vi "NI AO_test.vi"() -> ()   [LabVIEW 2019]
uses:
  <vilib>/Utility/error.llb/DialogType.ctl
  <vilib>/DAQmx/write.llb/DAQmx Write (Analog 1D Wfm NChan NSamp).vi
  <vilib>/DAQmx/create/channels.llb/DAQmx Create Channel (AO-Voltage-Basic).vi
  <vilib>/DAQmx/configure/timing.llb/DAQmx Timing (Sample Clock).vi
  <vilib>/DAQmx/configure/trigger.llb/DAQmx Start Trigger (Digital Edge).vi
  <vilib>/DAQmx/configure/trigger.llb/DAQmx Start Trigger (Time).vi
  <vilib>/DAQmx/configure/trigger.llb/DAQmx Start Trigger (Analog Edge).vi
  <vilib>/DAQmx/miscellaneous.llb/DAQmx Fill In Error Info.vi
  <resource>/objmgr/daqmx.rc
  <vilib>/measure/NI_MABase.lvlib
panel:
  in  "off time":dbl
  in  "offset":dbl=3.0 format="%#_13g"
  out "x-y":dbl
  in  "stop":bool
  in  "square wave duty cycle (%)":dbl=50.0 format="%0.2f"
  in  "Trigger Type":T1(tab)
  in  "Digital Start Trigger Edge":i32(ring)=10280 caption="Edge" items=["Rising"=10280, "Falling"=10171]
  in  "Digital Start Trigger Source":tag="/Dev1/PFI0" caption="Source"
  in  "Digital Pause Trigger Pause When":i32(ring)=10192 caption="Pause When" items=["High"=10192, "Low"=10214]
  in  "Digital Pause Trigger Source":tag="/Dev1/PFI0" caption="Source"
  in  "Analog Start Trigger Level":dbl caption="Level" format="%0.2f"
  in  "Analog Start Trigger Hysteresis":dbl caption="Hysteresis" format="%.2f"
  in  "Analog Start Trigger Slope":i32(ring)=10280 caption="Slope" items=["Rising"=10280, "Falling"=10171]
  in  "Analog Start Trigger Source":string="APFI0" caption="Source"
  in  "Analog Pause Trigger Source":string="APFI0" caption="Source"
  in  "Analog Pause Trigger Pause When":i32(ring)=10093 caption="Pause When" items=["Above Level"=10093, "Below Level"=10107]
  in  "Analog Pause Trigger Level":dbl caption="Level" format="%.2f"
  in  "When":timestamp
  in  "Select Time\nManually":bool
  out "Waveform Graph":waveform(dbl)[](graph)=[{"t0"=timestamp(0 s since 1904-01-01), "dt"=0.001, "Y"=[]}]
  in  "Output Array":T2(array[cluster])=[{"Waveform Type"=0, "Amplitude"=1.0, "Frequency"=10.0}] {"Frequency" format="%0.2p"; "Amplitude" format="%0.2p"; "Waveform Type" items=["Sine Wave", "Triangle Wave", "Square Wave", "Sawtooth Wave"]}
  in  "Number of Samples":i32=1000
  in  "Sample Rate":dbl=1000.0
  in  "Sample Clock Source":tag="OnboardClock"
  in  "Max Voltage":dbl=5.0
  in  "Min Voltage":dbl=-5.0
  in  "Physical Channel(s)":tag="Dev1/ao0"
  out "Actual Sample Rate":dbl=1000.0 format="%0.2f"
  # "To enable triggers, select a tab above, and configure the settings.\n\nNot all hardware supports all trigger types. Refer to your device documentation for more information."
  # "This trigger type is not supported in output tasks. \n\nRefer to your device documentation for more information on which triggers are supported."
  # "This trigger type is not supported in output tasks. \n\nRefer to your device documentation for more information on which triggers are supported."
  # "If time is not manually set, task will begin after 10 seconds"
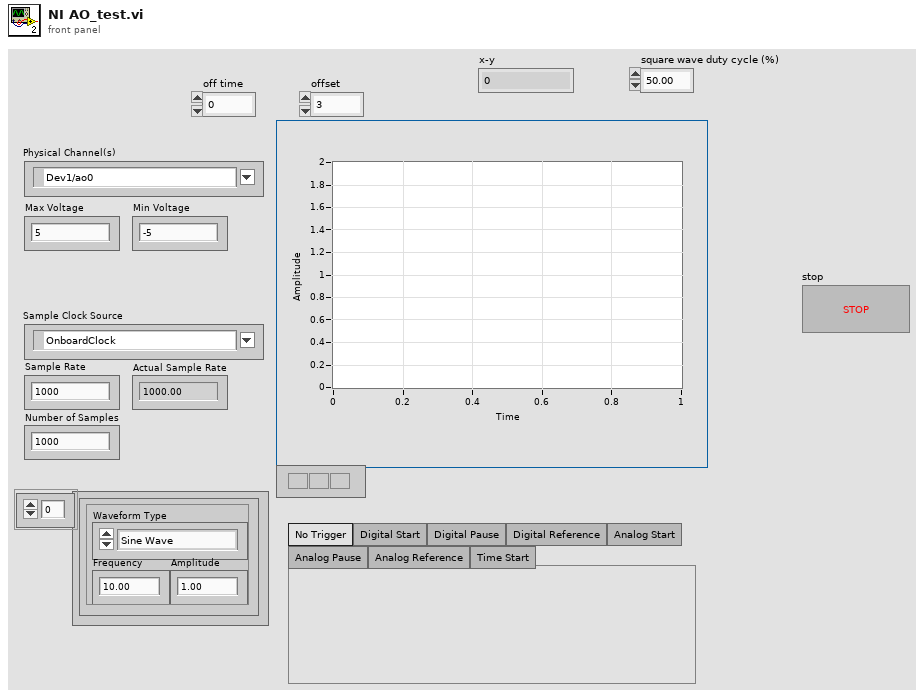
[diagram p1: front panel]
types:
  T1 = enum32{"No Trigger", "Digital Start", "Digital Pause", "Digital Reference", "Analog Start", "Analog Pause", "Analog Reference", "Time Start"}
  T2 = cluster{"Waveform Type":u16, "Amplitude":dbl, "Frequency":dbl}[]
  T3 = typedef "DialogType.ctl" = u16
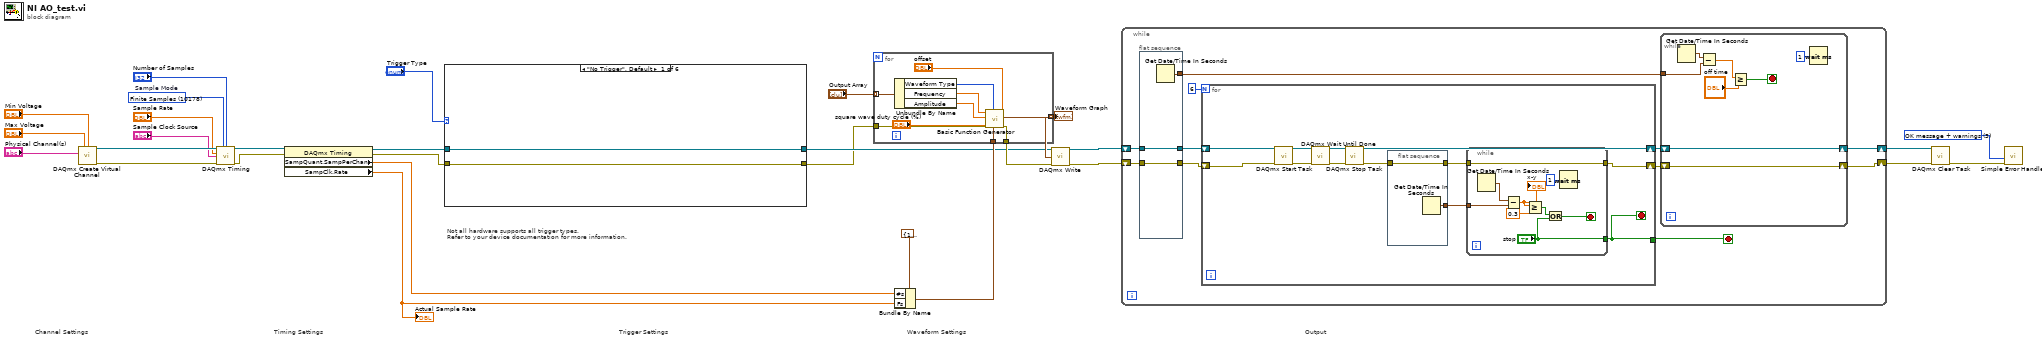
[diagram p0: block diagram]
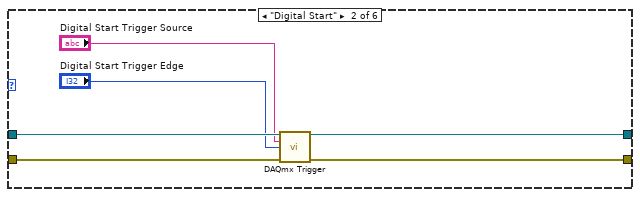
[diagram p2: hidden frame]
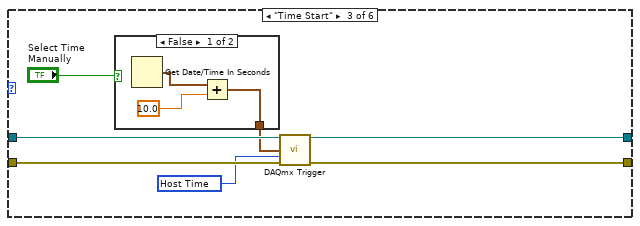
[diagram p3: hidden frame]
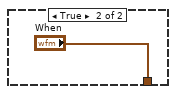
[diagram p4: hidden frame]
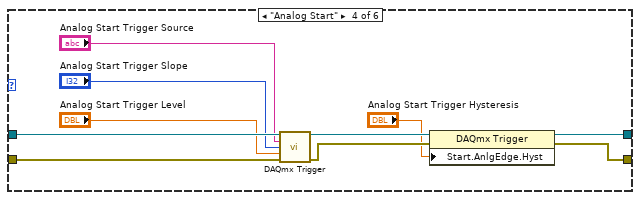
[diagram p5: hidden frame]
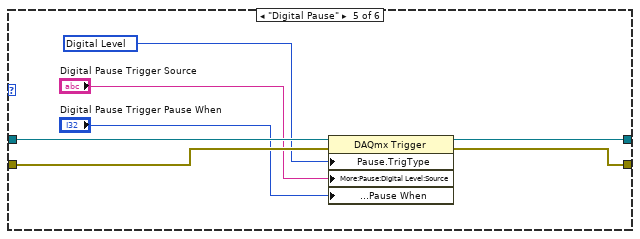
[diagram p6: hidden frame]
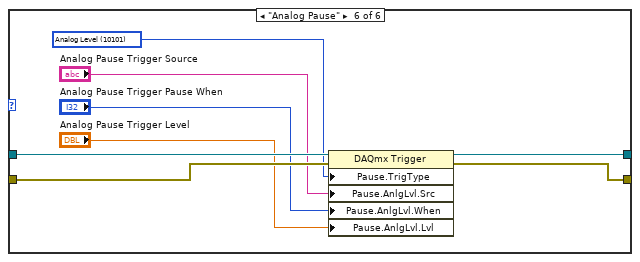
[diagram p7: hidden frame]
diagram:
  w6 = T3 3 items=["no dialog", "OK message", "continue or stop message", "OK message + warnings", "continue/stop + warnings"] ("type of dialog (OK msg:1)")
  w27 = 10178 items=["Finite Samples"=10178, "Continuous Samples"=10123, "Hardware Timed Single Point"=12522]  # Sample Mode
  # "Trigger Settings"
  # "Not all hardware supports all trigger types.\nRefer to your device documentation for more information."
  # "Output"
  # "Waveform Settings"
  # "Timing Settings"
  # "Channel Settings"
  n1 = call-poly <vilib>:"DAQmx Create Virtual Channel.vi"("maximum value"="Max Voltage", "minimum value"="Min Voltage", "physical channels"="Physical Channel(s)") -> ("task out"=w25:refnum<k21>, "error out"=w26:errorcluster)  [unwired: 11 in]
  n2 = call-poly <vilib>:"DAQmx Timing.vi"("task/channels in"=w25, "sample mode"=w27, "samples per channel"="Number of Samples", "rate"="Sample Rate", "source"="Sample Clock Source", "error in"=w26) -> ("task out"=w29:refnum<k21>, "error out"=w28:errorcluster)  [unwired: 8 in]
  n3 = property class="DAQmx Timing"(reference=w29, error in=w28) -> (reference out=w1:refnum<k21>, error out=w2:errorcluster, "SampQuant.SampPerChan"=w10:dbl, "SampClk.Rate"=w9:dbl)
  "Actual Sample Rate" <- w9
  n4 = case shown="\"No Trigger\", Default" "Trigger Type" {
    tunnel: w1 -> [w31 w37 w44 w58 w65 w73]
    tunnel: w2 -> [w30 w36 w43 w57 w62 w70]
    tunnel: [w31 w35 w42 w55 w64 w72] -> w4
    tunnel: [w30 w34 w41 w54 w63 w71] -> w3
    frame "No Trigger", Default {
    }
    frame "Digital Start" {
      n5 = call-poly <vilib>:"DAQmx Trigger.vi"("task/channels in"=w37, "source"="Digital Start Trigger Source", "edge"="Digital Start Trigger Edge", "error in"=w36) -> ("task out"=w35:refnum<k21>, "error out"=w34:errorcluster)  [unwired: 10 in]
    }
    frame "Time Start" {
      w40 = 16126 items=["Host Time"=16126, "I/O Device Time"=16127] ("timescale")
      n6 = case shown="False" "Select Time\nManually" {
        tunnel: [w46 "When"] -> w38
        frame False {
          n7 = Get Date/Time In Seconds() -> (seconds since 1Jan1904=w47:timestamp)
          n8 = Add(x=w47, y=10.0) -> (x+y=w46:timestamp)
        }
        frame True {
        }
      }
      n9 = call-poly <vilib>:"DAQmx Trigger.vi"("task/channels in"=w44, "when"=w38, "timescale"=w40, "error in"=w43) -> ("task out"=w42:refnum<k21>, "error out"=w41:errorcluster)  [unwired: 10 in]
    }
    frame "Analog Start" {
      n10 = call-poly <vilib>:"DAQmx Trigger.vi"("task/channels in"=w58, "source"="Analog Start Trigger Source", "slope"="Analog Start Trigger Slope", "level"="Analog Start Trigger Level", "error in"=w57) -> ("task out"=w53:refnum<k21>, "error out"=w52:errorcluster)  [unwired: 9 in]
      n11 = property class="DAQmx Trigger"(reference=w53, error in=w52, "Start.AnlgEdge.Hyst"="Analog Start Trigger Hysteresis") -> (reference out=w55:refnum<k21>, error out=w54:errorcluster)
    }
    frame "Digital Pause" {
      w61 = 10152 items=["Analog Level"=10101, "Analog Window"=10103, "Digital Level"=10152, "Digital Pattern"=10398, "None"=10230] ("Pause.TrigType")
      n12 = property class="DAQmx Trigger"(reference=w65, error in=w62, "Pause.TrigType"=w61, "More:Pause:Digital Level:Source"="Digital Pause Trigger Source", "More:Pause:Digital Level:Pause When"="Digital Pause Trigger Pause When") -> (reference out=w64:refnum<k21>, error out=w63:errorcluster)
    }
    frame "Analog Pause" {
      w69 = 10101 items=["Analog Level"=10101, "Analog Window"=10103, "Digital Level"=10152, "Digital Pattern"=10398, "None"=10230] ("Pause.TrigType")
      n13 = property class="DAQmx Trigger"(reference=w73, error in=w70, "Pause.TrigType"=w69, "Pause.AnlgLvl.Src"="Analog Pause Trigger Source", "Pause.AnlgLvl.When"="Analog Pause Trigger Pause When", "Pause.AnlgLvl.Lvl"="Analog Pause Trigger Level") -> (reference out=w72:refnum<k21>, error out=w71:errorcluster)
    }
  }
  n14 = Bundle By Name(cluster=cluster{"Fs":dbl, "#s":dbl} {"Fs"=1000.0, "#s"=1000.0} ("sampling info"), "#s"=w10, "Fs"=w9) -> (w17:cluster{"Fs":dbl, "#s":dbl})
  n15 = for {
    tunnel: w3 -> [w83]
    tunnel: w17 -> [w82]
    tunnel: [w81] -> w14
    tunnel: "Output Array" -> [w80] mode=indexing
    tunnel: [w76] -> w12 mode=indexing
    n16 = Unbundle By Name(w80) -> ("Waveform Type"=w79:u16, "Frequency"=w78:dbl, "Amplitude"=w77:dbl)
    n17 = call <vilib>:"Basic Function Generator.vi"("offset"="offset", "square wave duty cycle (%)"="square wave duty cycle (%)", "sampling info"=w82, "signal type"=w79, "error in (no error)"=w83, "amplitude"=w77, "frequency"=w78) -> ("error out"=w81:errorcluster, "signal out"=w76:waveform(dbl))  [unwired: 2 in, 1 out]
  }
  "Waveform Graph" <- w12
  n18 = call-poly <vilib>:"DAQmx Write.vi"("task/channels in"=w4, "data"=w12, "error in"=w14) -> ("task out"=w16:refnum<k21>, "error out"=w15:errorcluster)  [unwired: 10 in, 1 out]
  n19 = while {
    shift-right: [w89] -> w8
    shift-left: w16 -> [w92]
    shift-right: [w87] -> w7
    shift-left: w15 -> [w90]
    stop <- w94 stop-if-true
    n20 = flat-sequence {
      tunnel: [w105] -> w93
      tunnel: w92 -> [w105]
      tunnel: [w104] -> w91
      tunnel: w90 -> [w104]
      tunnel: [w103] -> w85
      frame #0 {
        n21 = Get Date/Time In Seconds() -> (seconds since 1Jan1904=w103:timestamp)
      }
    }
    n22 = for {
      N: 6 -> [_]
      tunnel: [w106] -> w94
      shift-right: [w113] -> w88
      shift-left: w93 -> [w117]
      shift-right: [w107] -> w86
      shift-left: w91 -> [w116]
      stop <- w106 stop-if-true
      n23 = call <vilib>:"DAQmx Start Task.vi"("task/channels in"=w117, "error in"=w116) -> ("task out"=w115:refnum<k21>, "error out"=w114:errorcluster)  [unwired: 12 in]
      n24 = call <vilib>:"DAQmx Wait Until Done.vi"("task/channels in"=w115, "error in"=w114) -> ("task out"=w112:refnum<k21>, "error out"=w111:errorcluster)  [unwired: 12 in]
      n25 = call <vilib>:"DAQmx Stop Task.vi"("task/channels in"=w112, "error in"=w111) -> ("task out"=w113:refnum<k21>, "error out"=w109:errorcluster)  [unwired: 12 in]
      n26 = flat-sequence {
        tunnel: [w119] -> w110
        tunnel: w109 -> [w119]
        tunnel: [w118] -> w108
        frame #0 {
          n27 = Get Date/Time In Seconds() -> (seconds since 1Jan1904=w118:timestamp)
        }
      }
      n28 = while {
        tunnel: [w128] -> w107
        tunnel: w110 -> [w128]
        tunnel: w108 -> [w126]
        tunnel: ["stop"] -> w106
        stop <- w122 stop-if-true
        n29 = Get Date/Time In Seconds() -> (seconds since 1Jan1904=w127:timestamp)
        n30 = Subtract(x=w127, y=w126) -> (x-y=w125:dbl)
        "x-y" <- w125
        n31 = Greater Or Equal?(x=w125, y=0.3) -> (x >= y?=w123:bool)
        n32 = Or(x=w123, y="stop") -> (x .or. y?=w122:bool)
        n33 = Wait (ms)(milliseconds to wait=u32 1) -> ()  [unwired: 1 out]
      }
    }
    n34 = while {
      shift-right: [w102] -> w89
      shift-left: w88 -> [w102]
      shift-right: [w101] -> w87
      shift-left: w86 -> [w101]
      tunnel: w85 -> [w99]
      stop <- w96 stop-if-true
      n35 = Get Date/Time In Seconds() -> (seconds since 1Jan1904=w100:timestamp)
      n36 = Subtract(x=w100, y=w99) -> (x-y=w98:dbl)
      n37 = Greater Or Equal?(x=w98, y="off time") -> (x >= y?=w96:bool)
      n38 = Wait (ms)(milliseconds to wait=u32 1) -> ()  [unwired: 1 out]
    }
  }
  n39 = call <vilib>:"DAQmx Clear Task.vi"("task in"=w8, "error in"=w7) -> ("error out"=w24:errorcluster)  [unwired: 13 in]
  n40 = call <vilib>:"Simple Error Handler.vi"("type of dialog (OK msg:1)"=w6, "error in (no error)"=w24) -> ()  [unwired: 3 in, 5 out]
